vi "pumonarytesting_strain.vi"() -> ()   [LabVIEW 2014]
uses:
  <vilib>/vision/NI_Vision_Development_Module.lvlib
  <instrlib>/KD Scientific 2XX Series/KD Scientific 2XX Series.lvlib
panel:
  in  "Number of Cycles":i32
  in  "Min Pressure":dbl
  in  "Max Pressure":dbl
  out "Status":T1
  in  "stop 2":bool
  out "Delivered Volume":dbl
  out "Units":string
  in  "Baud Rate (9600)":u32(ring)=9600 items=["300"=300, "1200"=1200, "2400"=2400, "4800"=4800, "9600"=9600]
  in  "Withdrawal Settings":T2={"Flow Rate (5)"=5.0, "Volume (10)"=10.0, "Volume Units (ml)"=enum."milliliters (ml)", "Rate Units (ml/min.)"=enum."milliliters per minute (ml/min.)"} {"Volume (10)" format="%#.3g"}
  in  "Diameter (8.75 mm)":dbl=8.75
  in  "Infusion Settings":T2={"Flow Rate (5)"=5.0, "Volume (10)"=10.0, "Volume Units (ml)"=enum."milliliters (ml)", "Rate Units (ml/min.)"=enum."milliliters per minute (ml/min.)"}
  in  "Address (0)":i32 format="%0.0f"
  in  "error in (no error)":errorcluster
  in  "VISA resource name":refnum<visa-resource-name>="COM1"
  in  "stop 4":bool
  in  "stop":bool
  out "Image":T3(plugin-control)
  out "Particle Measurements (Pixels) (Particle Analysis 1)":dbl[][](array[numeric]) format="%.2f"
  out "subarray":dbl[](array[numeric])
  out "The diameter":dbl[](array[numeric])
  in  "stop (F)":bool
  out "Data from Transducer":dynamicdata(graph) caption="Voltage from Transducer V"
  out "Voltage from pressure transducer":dbl[](array[numeric])
  out "Pressure mm Hg":dbl[](graph)
  in  "Calibration factor":dbl[](array[numeric])
  in  "Zero Error":dbl[](array[numeric])
  out "pressure mm Hg":dbl[](array[numeric])
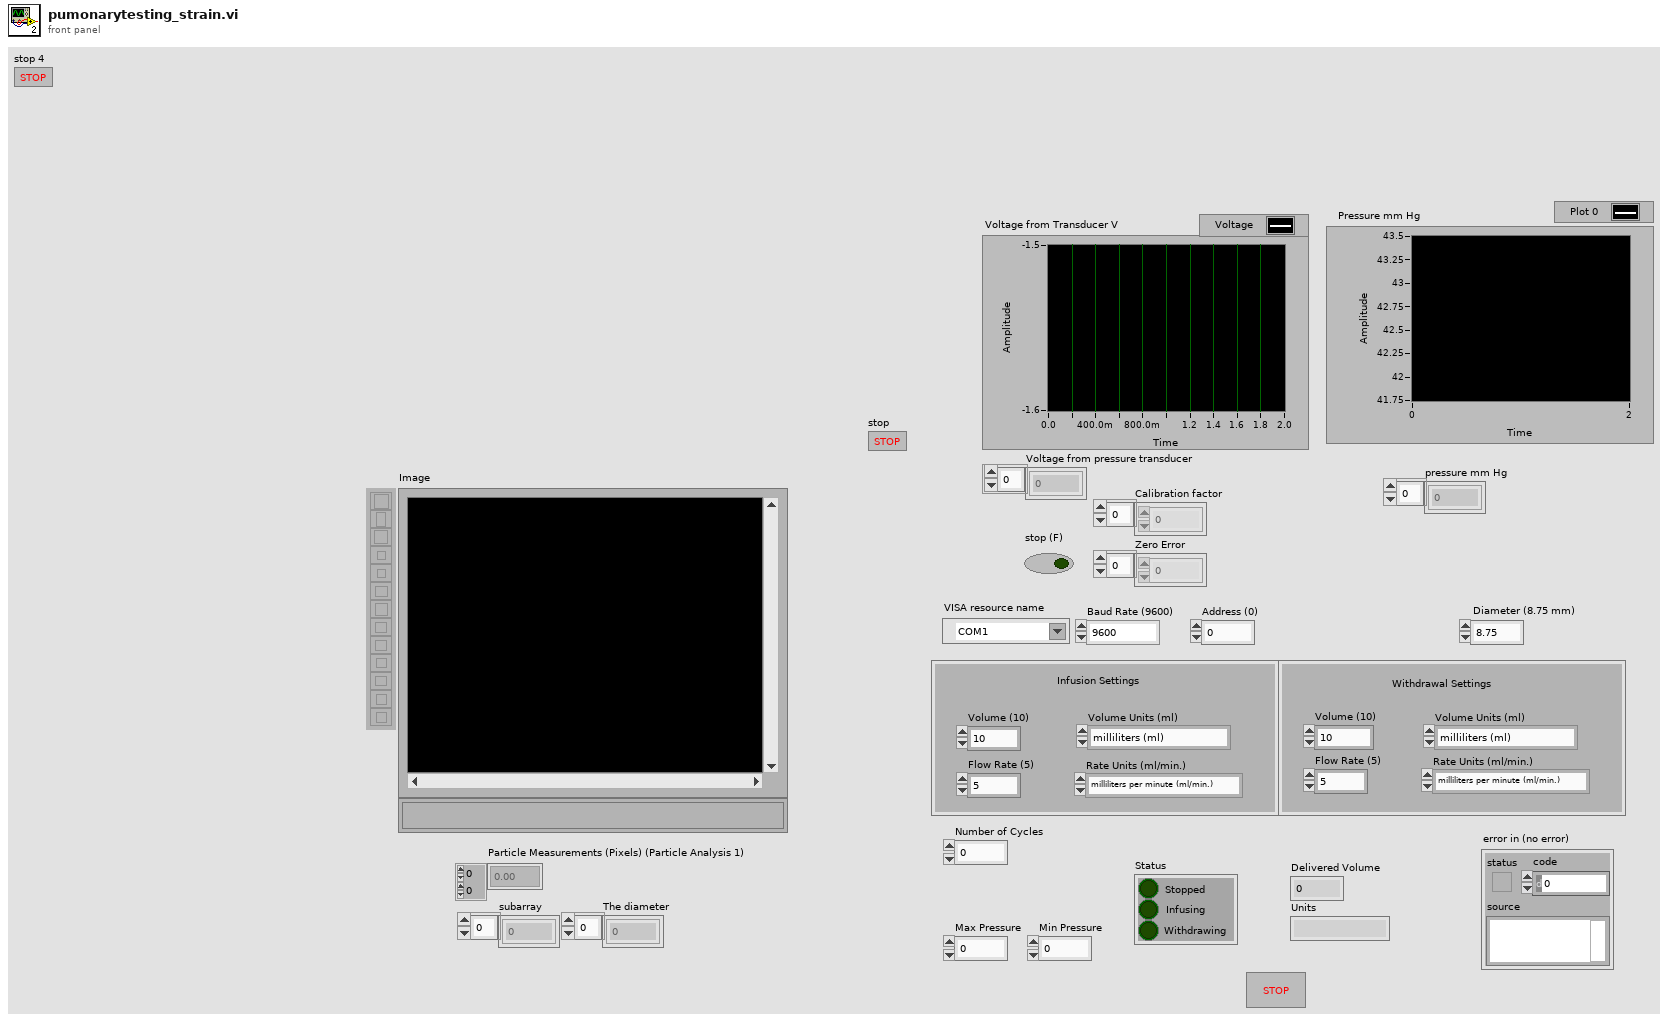
[diagram p1: front panel]
types:
  T1 = cluster{"Stopped":bool, "Infusing":bool, "Withdrawing":bool}
  T2 = cluster{"Flow Rate (5)":dbl, "Volume (10)":dbl, "Volume Units (ml)":enum16{"milliliters (ml)", "microliters (ul)"}, "Rate Units (ml/min.)":enum16{"milliliters per minute (ml/min.)", "milliliters per hour (ml/hr.)", "microliters per minute (ul/min.)", "microliters per hour (ul/hr.)"}}
  T3 = typedef "IMAQ Image.ctl" = refnum<image>
  T4 = typedef "Board Id" = u8
  T5 = typedef "ROI Descriptor" = cluster{"Global Rectangle":i32[], "Contours":cluster{"ID":enum32{"External", "Internal"}, "Type":u32, "Coordinates":i32[]}[]}
  T6 = enum16{"milliliters per minute (ml/min.)", "milliliters per hour (ml/hr.)", "microliters per minute (ul/min.)", "microliters per hour (ul/hr.)"}
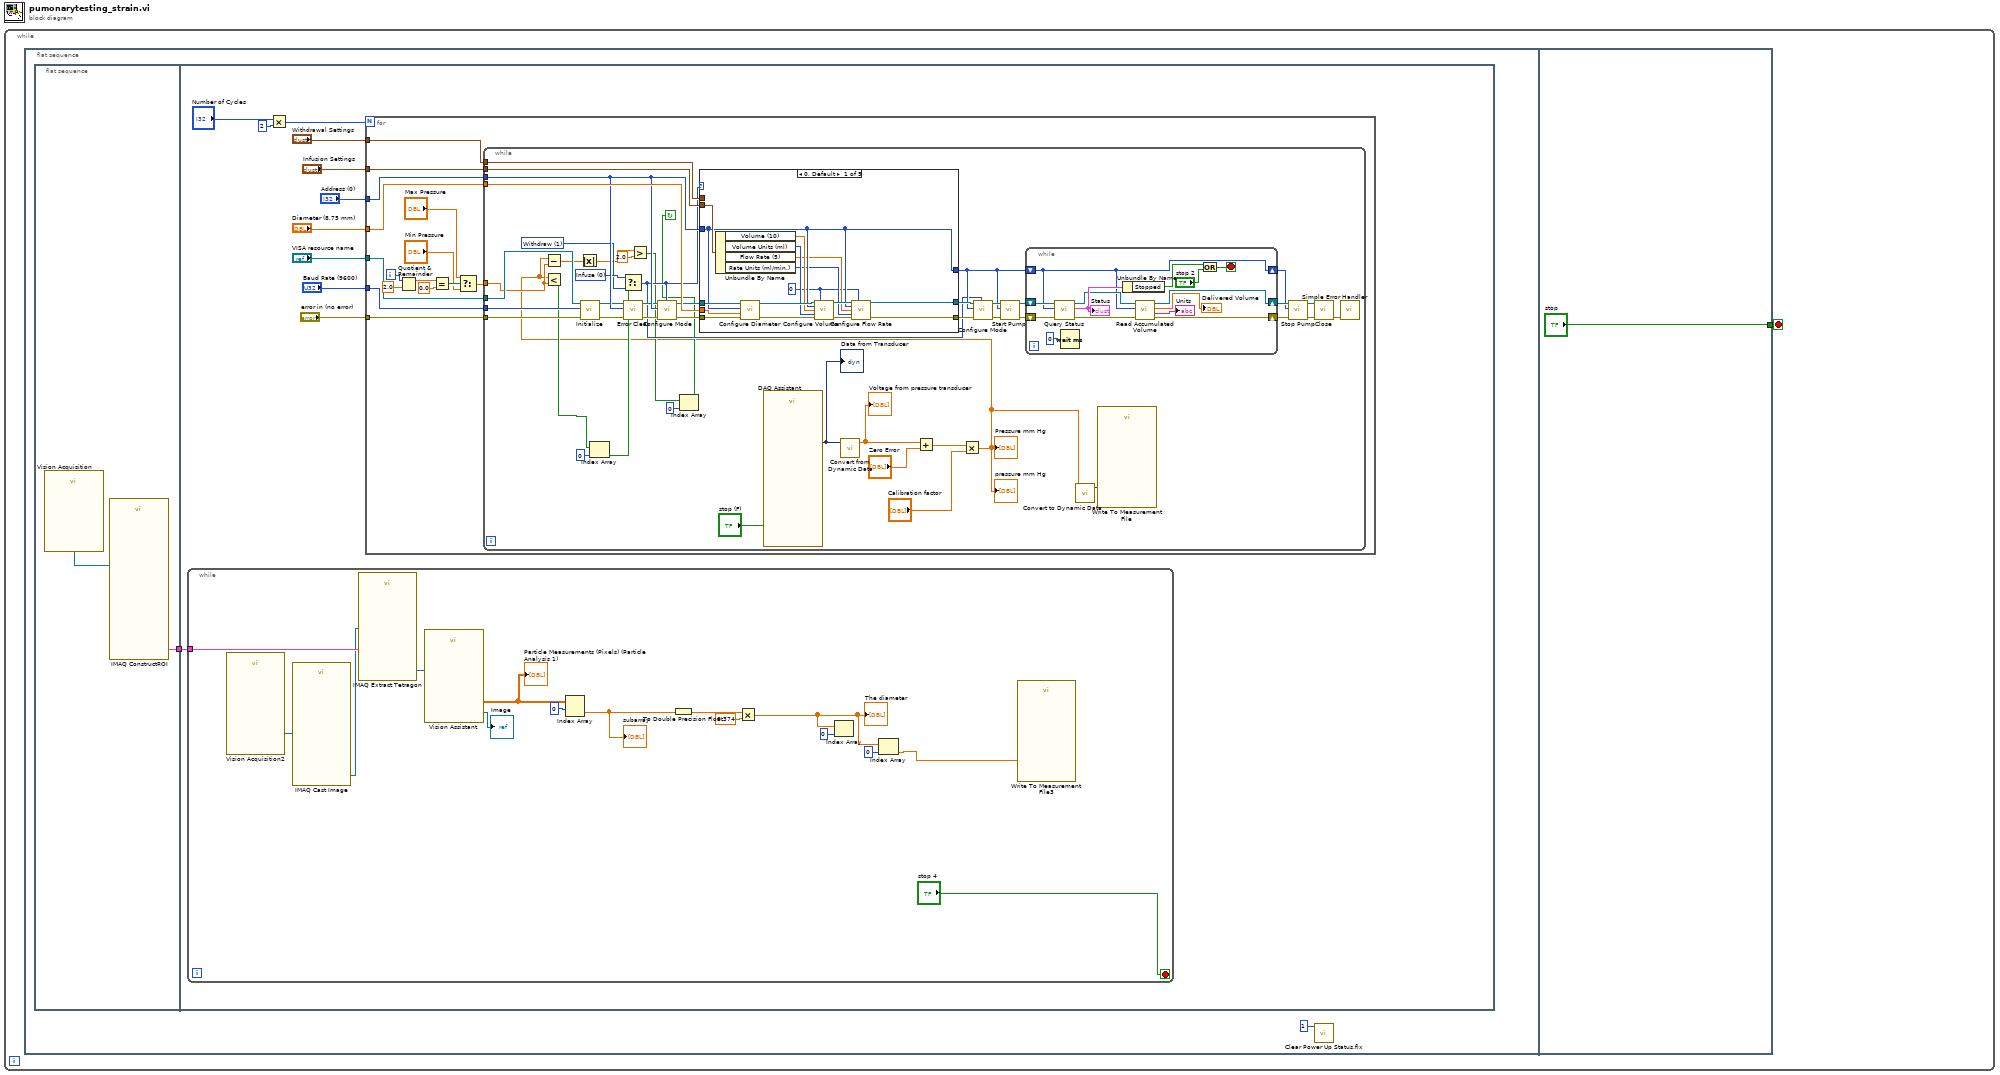
[diagram p0: block diagram]
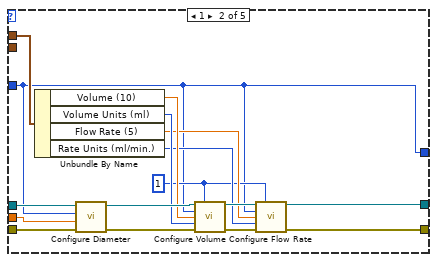
[diagram p2: hidden frame]
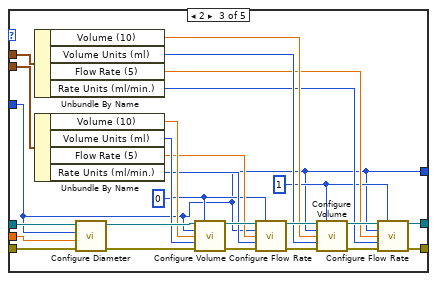
[diagram p3: hidden frame]
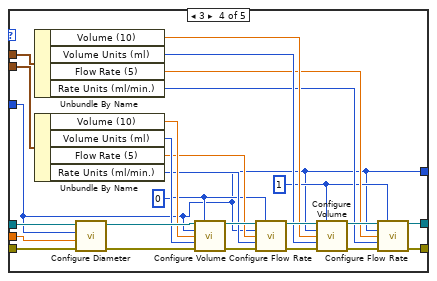
[diagram p4: hidden frame]
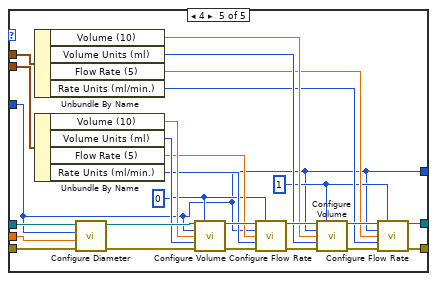
[diagram p5: hidden frame]
diagram:
  n1 = while {
    stop <- w1 stop-if-true
    n2 = flat-sequence {
      tunnel: ["stop"] -> w1
      frame #0 {
        n3 = flat-sequence {
          tunnel: [w4] -> w3
          tunnel: w3 -> [w16]
          frame #0 {
            n4 = call "Vision Acquisition"() -> ("Image Out"=w5:T3)  [unwired: 26 in, 1 out]
            n5 = call "IMAQ ConstructROI"("Image"=w5) -> ("ROI Descriptor Out"=w4:T5)  [unwired: 7 in, 3 out]
          }
          frame #1 {
            n6 = while {
              tunnel: w16 -> [w217]
              stop <- "stop 4" stop-if-true
              n7 = call "Vision Acquisition2"() -> ("Image Out"=w207:T3)  [unwired: 25 in, 2 out]
              n8 = call "IMAQ Cast Image"("Image Src"=w207) -> ("Image Dst Out"=w214:T3)  [unwired: 9 in, 1 out]
              n9 = call-poly "IMAQ Extract Tetragon"("ROI Descriptor"=w217, "Image Src"=w214) -> ("Image Dst Out"=w215:T3)  [unwired: 8 in, 1 out]
              n10 = call "Vision Assistant"("Image In"=w215) -> ("Image Out"=→"Image":T3, "Particle Measurements (Pixels) (Particle Analysis 1)"=w213:dbl[][])  [unwired: 23 in, 2 out]
              "Particle Measurements (Pixels) (Particle Analysis 1)" <- w213
              n11 = Index Array(array=w213, index (row)=0) -> (element=w211:dbl[])  [unwired: 1 in]
              "subarray" <- w211
              n12 = To Double Precision Float(number=w211) -> (double precision float=w210:dbl[])
              n13 = Multiply(x=w210, y=0.374) -> (x*y=w204:dbl[])
              "The diameter" <- w204
              n14 = Index Array(array=w204, index=0) -> ()  [unwired: 1 out]
              n15 = Index Array(array=w204, index=0) -> (element=w203:dbl)
              n16 = call "Write To Measurement File3"("Signals"=w203) -> ()  [unwired: 16 in, 3 out]
            }
            n17 = Multiply(x="Number of Cycles", y=2) -> (x*y=w15:i32)
            n18 = for {
              N: w15 -> [_]
              tunnel: "VISA resource name" -> [w31]
              tunnel: "error in (no error)" -> [w30]
              tunnel: "Infusion Settings" -> [w29]
              tunnel: "Withdrawal Settings" -> [w28]
              tunnel: "Diameter (8.75 mm)" -> [w27]
              tunnel: "Baud Rate (9600)" -> [w26]
              tunnel: "Address (0)" -> [w25]
              i -> [w23]
              n19 = Quotient & Remainder(x=w23, y=2.0) -> (x-y*floor(x/y)=w21:dbl)  [unwired: 1 out]
              n20 = Equal?(x=w21, y=0.0) -> (x = y?=w20:bool)
              n21 = Select(t="Max Pressure", s=w20, f="Min Pressure") -> (s? t:f=w17:dbl)
              n22 = while {
                tunnel: w31 -> [w78]
                tunnel: w30 -> [w77]
                tunnel: w29 -> [w76]
                tunnel: w28 -> [w75]
                tunnel: w27 -> [w74]
                tunnel: w26 -> [w73]
                tunnel: w25 -> [w72]
                tunnel: w17 -> [w49]
                stop <- w34 continue-if-true
                w51 = u16 1 items=["Withdraw"=1]
                w52 = u16 0 items=["Infuse"] ("Mode (infuse)")
                n23 = call <instrlib>:"Initialize.vi"("error in (no error)"=w77, "Baud Rate (9600)"=w73, "VISA resource name"=w78) -> ("error out"=w54:errorcluster, "VISA resource name out"=w53:refnum<visa-resource-name>)  [unwired: 7 in]
                n24 = call <instrlib>:"Error Clear.vi"("error in (no error)"=w54, "Address (0)"=w72, "VISA resource name"=w53) -> ("error out"=w55:errorcluster, "VISA resource name out"=w56:refnum<visa-resource-name>)  [unwired: 6 in, 1 out]
                n25 = call "DAQ Assistant"("stop (F)"="stop (F)") -> ("data"=w40:dynamicdata)  [unwired: 15 in, 3 out]
                "Data from Transducer" <- w40
                n26 = call "Convert from Dynamic Data"("Dynamic Data Type"=w40) -> ("Array"=w43:dbl[])  [unwired: 3 in]
                "Voltage from pressure transducer" <- w43
                n27 = Add(x=w43, y="Zero Error") -> (x+y=w41:dbl[])
                n28 = Multiply(x=w41, y="Calibration factor") -> (x*y=w33:dbl[])
                "Pressure mm Hg" <- w33
                "pressure mm Hg" <- w33
                n29 = Subtract(x=w33, y=w49) -> (x-y=w48:dbl[])
                n30 = Less?(x=w33, y=w49) -> (x < y?=w39:bool[])
                n31 = Absolute Value(x=w48) -> (abs(x)=w47:dbl[])
                n32 = Index Array(array=w39, index=0) -> (element=w37:bool)
                n33 = Select(t=w52, s=w37, f=w51) -> (s? t:f=w50:u16)
                n34 = Greater?(x=w47, y=2.0) -> (0:w36:bool[])
                n35 = call <instrlib>:"Configure Mode.vi"("Mode (infuse)"=w50, "error in (no error)"=w55, "Address (0)"=w72, "VISA resource name"=w56) -> ("error out"=w58:errorcluster, "VISA resource name out"=w57:refnum<visa-resource-name>)  [unwired: 6 in]
                n36 = Index Array(array=w36, index=0) -> (element=w34:bool)
                n37 = case shown="0, Default" w50 {
                  tunnel: w76 -> [w88 _ w136 w162 w188]
                  tunnel: w75 -> [_ w110 w135 w161 w187]
                  tunnel: w57 -> [w94 w109 w134 w160 w186]
                  tunnel: w58 -> [w93 w105 w133 w159 w185]
                  tunnel: w74 -> [w87 w101 w116 w142 w168]
                  tunnel: [w86 w95 w111 w137 w163] -> w59
                  tunnel: w72 -> [w86 w95 w111 w137 w163]
                  tunnel: [w81 w106 w113 w139 w165] -> w63
                  tunnel: [w80 w102 w112 w138 w164] -> w62
                  frame 0, Default {
                    w79 = 0
                    n38 = Unbundle By Name(w88) -> ("Volume (10)"=w85:dbl, "Volume Units (ml)"=w84:enum16{"milliliters (ml)", "microliters (ul)"}, "Flow Rate (5)"=w83:dbl, "Rate Units (ml/min.)"=w82:T6)
                    n39 = call <instrlib>:"Configure Diameter.vi"("error in (no error)"=w93, "Diameter (8.75 mm)"=w87, "Address (0)"=w86, "VISA resource name"=w94) -> ("error out"=w91:errorcluster, "VISA resource name out"=w92:refnum<visa-resource-name>)  [unwired: 6 in]
                    n40 = call <instrlib>:"Configure Volume.vi"("VISA resource name"=w92, "Mode (infuse)"=w79, "Address (0)"=w86, "Volume (100)"=w85, "Units (0: milliliters)"=w84, "error in (no error)"=w91) -> ("VISA resource name out"=w90:refnum<visa-resource-name>, "error out"=w89:errorcluster)  [unwired: 8 in]
                    n41 = call <instrlib>:"Configure Flow Rate.vi"("VISA resource name"=w90, "Mode (infuse)"=w79, "Address (0)"=w86, "Flow Rate (5)"=w83, "Units (0: milliliters per minute)"=w82, "error in (no error)"=w89) -> ("VISA resource name out"=w81:refnum<visa-resource-name>, "error out"=w80:errorcluster)  [unwired: 8 in]
                  }
                  frame 1 {
                    w96 = 1
                    n42 = Unbundle By Name(w110) -> ("Volume (10)"=w100:dbl, "Volume Units (ml)"=w99:enum16{"milliliters (ml)", "microliters (ul)"}, "Flow Rate (5)"=w98:dbl, "Rate Units (ml/min.)"=w97:T6)
                    n43 = call <instrlib>:"Configure Diameter.vi"("error in (no error)"=w105, "Diameter (8.75 mm)"=w101, "Address (0)"=w95, "VISA resource name"=w109) -> ("error out"=w104:errorcluster, "VISA resource name out"=w108:refnum<visa-resource-name>)  [unwired: 6 in]
                    n44 = call <instrlib>:"Configure Volume.vi"("VISA resource name"=w108, "Mode (infuse)"=w96, "Address (0)"=w95, "Volume (100)"=w100, "Units (0: milliliters)"=w99, "error in (no error)"=w104) -> ("VISA resource name out"=w107:refnum<visa-resource-name>, "error out"=w103:errorcluster)  [unwired: 8 in]
                    n45 = call <instrlib>:"Configure Flow Rate.vi"("VISA resource name"=w107, "Mode (infuse)"=w96, "Address (0)"=w95, "Flow Rate (5)"=w98, "Units (0: milliliters per minute)"=w97, "error in (no error)"=w103) -> ("VISA resource name out"=w106:refnum<visa-resource-name>, "error out"=w102:errorcluster)  [unwired: 8 in]
                  }
                  frame 2 {
                    w114 = 1
                    w115 = 0
                    n46 = Unbundle By Name(w135) -> ("Volume (10)"=w120:dbl, "Volume Units (ml)"=w119:enum16{"milliliters (ml)", "microliters (ul)"}, "Flow Rate (5)"=w118:dbl, "Rate Units (ml/min.)"=w117:T6)
                    n47 = Unbundle By Name(w136) -> ("Volume (10)"=w124:dbl, "Volume Units (ml)"=w123:enum16{"milliliters (ml)", "microliters (ul)"}, "Flow Rate (5)"=w122:dbl, "Rate Units (ml/min.)"=w121:T6)
                    n48 = call <instrlib>:"Configure Diameter.vi"("error in (no error)"=w133, "Diameter (8.75 mm)"=w116, "Address (0)"=w111, "VISA resource name"=w134) -> ("error out"=w128:errorcluster, "VISA resource name out"=w132:refnum<visa-resource-name>)  [unwired: 6 in]
                    n49 = call <instrlib>:"Configure Volume.vi"("VISA resource name"=w132, "Mode (infuse)"=w115, "Address (0)"=w111, "Volume (100)"=w124, "Units (0: milliliters)"=w123, "error in (no error)"=w128) -> ("VISA resource name out"=w131:refnum<visa-resource-name>, "error out"=w127:errorcluster)  [unwired: 8 in]
                    n50 = call <instrlib>:"Configure Flow Rate.vi"("VISA resource name"=w131, "Mode (infuse)"=w115, "Address (0)"=w111, "Flow Rate (5)"=w122, "Units (0: milliliters per minute)"=w121, "error in (no error)"=w127) -> ("VISA resource name out"=w130:refnum<visa-resource-name>, "error out"=w126:errorcluster)  [unwired: 8 in]
                    n51 = call <instrlib>:"Configure Volume.vi"("VISA resource name"=w130, "Mode (infuse)"=w114, "Address (0)"=w111, "Volume (100)"=w120, "Units (0: milliliters)"=w119, "error in (no error)"=w126) -> ("VISA resource name out"=w129:refnum<visa-resource-name>, "error out"=w125:errorcluster)  [unwired: 8 in]
                    n52 = call <instrlib>:"Configure Flow Rate.vi"("VISA resource name"=w129, "Mode (infuse)"=w114, "Address (0)"=w111, "Flow Rate (5)"=w118, "Units (0: milliliters per minute)"=w117, "error in (no error)"=w125) -> ("VISA resource name out"=w113:refnum<visa-resource-name>, "error out"=w112:errorcluster)  [unwired: 8 in]
                  }
                  frame 3 {
                    w140 = 1
                    w141 = 0
                    n53 = Unbundle By Name(w161) -> ("Volume (10)"=w146:dbl, "Volume Units (ml)"=w145:enum16{"milliliters (ml)", "microliters (ul)"}, "Flow Rate (5)"=w144:dbl, "Rate Units (ml/min.)"=w143:T6)
                    n54 = Unbundle By Name(w162) -> ("Volume (10)"=w150:dbl, "Volume Units (ml)"=w149:enum16{"milliliters (ml)", "microliters (ul)"}, "Flow Rate (5)"=w148:dbl, "Rate Units (ml/min.)"=w147:T6)
                    n55 = call <instrlib>:"Configure Diameter.vi"("error in (no error)"=w159, "Diameter (8.75 mm)"=w142, "Address (0)"=w137, "VISA resource name"=w160) -> ("error out"=w154:errorcluster, "VISA resource name out"=w158:refnum<visa-resource-name>)  [unwired: 6 in]
                    n56 = call <instrlib>:"Configure Volume.vi"("VISA resource name"=w158, "Mode (infuse)"=w141, "Address (0)"=w137, "Volume (100)"=w150, "Units (0: milliliters)"=w149, "error in (no error)"=w154) -> ("VISA resource name out"=w157:refnum<visa-resource-name>, "error out"=w153:errorcluster)  [unwired: 8 in]
                    n57 = call <instrlib>:"Configure Flow Rate.vi"("VISA resource name"=w157, "Mode (infuse)"=w141, "Address (0)"=w137, "Flow Rate (5)"=w148, "Units (0: milliliters per minute)"=w147, "error in (no error)"=w153) -> ("VISA resource name out"=w156:refnum<visa-resource-name>, "error out"=w152:errorcluster)  [unwired: 8 in]
                    n58 = call <instrlib>:"Configure Volume.vi"("VISA resource name"=w156, "Mode (infuse)"=w140, "Address (0)"=w137, "Volume (100)"=w146, "Units (0: milliliters)"=w145, "error in (no error)"=w152) -> ("VISA resource name out"=w155:refnum<visa-resource-name>, "error out"=w151:errorcluster)  [unwired: 8 in]
                    n59 = call <instrlib>:"Configure Flow Rate.vi"("VISA resource name"=w155, "Mode (infuse)"=w140, "Address (0)"=w137, "Flow Rate (5)"=w144, "Units (0: milliliters per minute)"=w143, "error in (no error)"=w151) -> ("VISA resource name out"=w139:refnum<visa-resource-name>, "error out"=w138:errorcluster)  [unwired: 8 in]
                  }
                  frame 4 {
                    w166 = 1
                    w167 = 0
                    n60 = Unbundle By Name(w187) -> ("Volume (10)"=w172:dbl, "Volume Units (ml)"=w171:enum16{"milliliters (ml)", "microliters (ul)"}, "Flow Rate (5)"=w170:dbl, "Rate Units (ml/min.)"=w169:T6)
                    n61 = Unbundle By Name(w188) -> ("Volume (10)"=w176:dbl, "Volume Units (ml)"=w175:enum16{"milliliters (ml)", "microliters (ul)"}, "Flow Rate (5)"=w174:dbl, "Rate Units (ml/min.)"=w173:T6)
                    n62 = call <instrlib>:"Configure Diameter.vi"("error in (no error)"=w185, "Diameter (8.75 mm)"=w168, "Address (0)"=w163, "VISA resource name"=w186) -> ("error out"=w180:errorcluster, "VISA resource name out"=w184:refnum<visa-resource-name>)  [unwired: 6 in]
                    n63 = call <instrlib>:"Configure Volume.vi"("VISA resource name"=w184, "Mode (infuse)"=w167, "Address (0)"=w163, "Volume (100)"=w176, "Units (0: milliliters)"=w175, "error in (no error)"=w180) -> ("VISA resource name out"=w183:refnum<visa-resource-name>, "error out"=w179:errorcluster)  [unwired: 8 in]
                    n64 = call <instrlib>:"Configure Flow Rate.vi"("VISA resource name"=w183, "Mode (infuse)"=w167, "Address (0)"=w163, "Flow Rate (5)"=w174, "Units (0: milliliters per minute)"=w173, "error in (no error)"=w179) -> ("VISA resource name out"=w182:refnum<visa-resource-name>, "error out"=w178:errorcluster)  [unwired: 8 in]
                    n65 = call <instrlib>:"Configure Volume.vi"("VISA resource name"=w182, "Mode (infuse)"=w166, "Address (0)"=w163, "Volume (100)"=w172, "Units (0: milliliters)"=w171, "error in (no error)"=w178) -> ("VISA resource name out"=w181:refnum<visa-resource-name>, "error out"=w177:errorcluster)  [unwired: 8 in]
                    n66 = call <instrlib>:"Configure Flow Rate.vi"("VISA resource name"=w181, "Mode (infuse)"=w166, "Address (0)"=w163, "Flow Rate (5)"=w170, "Units (0: milliliters per minute)"=w169, "error in (no error)"=w177) -> ("VISA resource name out"=w165:refnum<visa-resource-name>, "error out"=w164:errorcluster)  [unwired: 8 in]
                  }
                }
                n67 = call <instrlib>:"Configure Mode.vi"("Mode (infuse)"=w50, "error in (no error)"=w62, "Address (0)"=w59, "VISA resource name"=w63) -> ("error out"=w60:errorcluster, "VISA resource name out"=w61:refnum<visa-resource-name>)  [unwired: 6 in]
                n68 = call <instrlib>:"Start Pump.vi"("error in (no error)"=w60, "Address (0)"=w59, "VISA resource name"=w61) -> ("error out"=w70:errorcluster, "VISA resource name out"=w71:refnum<visa-resource-name>)  [unwired: 7 in]
                n69 = while {
                  shift-right: [w191] -> w67
                  shift-left: w59 -> [w191]
                  shift-right: [w193] -> w69
                  shift-left: w71 -> [w199]
                  shift-right: [w192] -> w68
                  shift-left: w70 -> [w200]
                  stop <- w197 stop-if-true
                  n70 = call <instrlib>:"Query Status.vi"("error in (no error)"=w200, "Address (0)"=w191, "VISA resource name"=w199) -> ("error out"=w202:errorcluster, "Status"=w198:T1, "VISA resource name out"=w194:refnum<visa-resource-name>)  [unwired: 6 in]
                  "Status" <- w198
                  n71 = Wait (ms)(milliseconds to wait=u32 0) -> ()  [unwired: 1 out]
                  n72 = Unbundle By Name(w198) -> ("Stopped"=w196:bool)
                  n73 = call <instrlib>:"Read Accumulated Volume.vi"("error in (no error)"=w202, "Address (0)"=w191, "VISA resource name"=w194) -> ("error out"=w192:errorcluster, "Units"=→"Units":string, "Delivered Volume"=→"Delivered Volume":dbl, "VISA resource name out"=w193:refnum<visa-resource-name>)  [unwired: 5 in]
                  n74 = Or(x=w196, y="stop 2") -> (x .or. y?=w197:bool)
                }
                n75 = call "Convert to Dynamic Data"("Array"=w33) -> ("Dynamic Data Type"=w32:dynamicdata)  [unwired: 3 in]
                n76 = call "Write To Measurement File"("Signals"=w32) -> ()  [unwired: 16 in, 3 out]
                n77 = call <instrlib>:"Stop Pump.vi"("error in (no error)"=w68, "Address (0)"=w67, "VISA resource name"=w69) -> ("error out"=w65:errorcluster, "VISA resource name out"=w64:refnum<visa-resource-name>)  [unwired: 7 in]
                n78 = call <instrlib>:"Close.vi"("error in (no error)"=w65, "VISA resource name"=w64) -> ("error out"=w66:errorcluster)  [unwired: 9 in]
                n79 = call <vilib>:"Simple Error Handler.vi"("error in (no error)"=w66) -> ()  [unwired: 4 in, 5 out]
              }
            }
          }
        }
        n80 = call <vilib>:"Clear Power Up Status.flx"("Board ID"=T4 1) -> ()  [unwired: 6 in, 2 out]
      }
      frame #1 {
      }
    }
  }
